vi "Create.vi"(0 "ClassWriter":refnum<class "ClassWriter.lvclass">, 5 "error in (no error)":errorcluster) -> (14 "ClassWriter":refnum<class "ClassWriter.lvclass">, 19 "error out":errorcluster)   [LabVIEW 2012, in "ClassWriter.lvclass"]
doc: "Creates and initializes a new ClassWriter object.\n\nThis object should be destroyed using a ClassWriter destructor VI.\n\n[GOOP 2.0.16]"
uses:
  <resource>/Framework/Providers/Open_GDS/ClassProviders/Provider_BaseClassInterface/ClassWriter_class/ClassWriter.lvclass
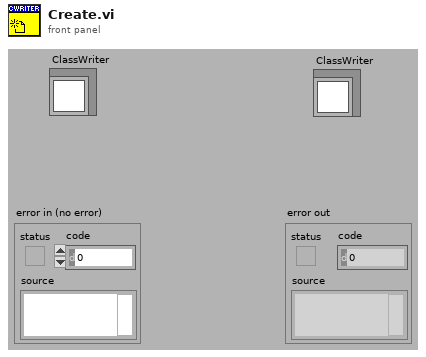
[diagram p1: front panel]
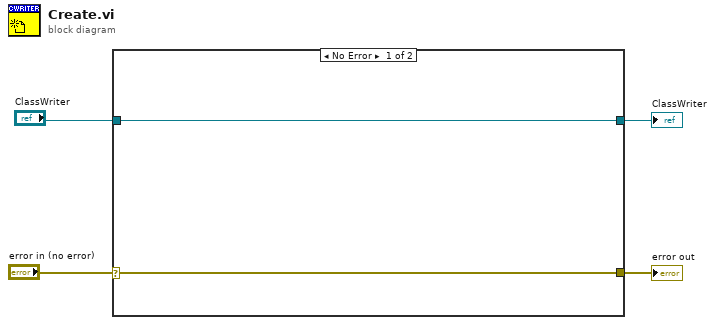
[diagram p0: block diagram]
diagram:
  n1 = case shown="No Error" "error in (no error)" {
    selector: "error in (no error)" -> [w6 w8]
    tunnel: [w5 w7] -> w4
    tunnel: [w6 w8] -> w3
    tunnel: "ClassWriter" -> [w5 w7]
    frame No Error {
    }
    frame Error {
    }
  }
  "error out" <- w3
  "ClassWriter" <- w4
